vi "NavX Zero Yaw.vi"(11 "Reset NavX Yaw":bool=TRUE) -> ()   [LabVIEW 2014]
uses:
  Navx data.vi
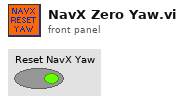
[diagram p1: front panel]
types:
  T1 = typedef "navX-MXP IMU.lvlib/navX YPRH Data.ctl" = cluster{"Yaw":dbl, "Pitch":dbl, "Roll":dbl, "Heading":dbl}
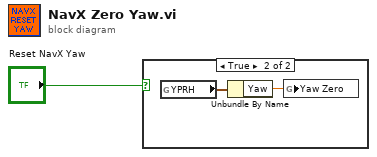
[diagram p0: block diagram]
diagram:
  n1 = case shown="True" "Reset NavX Yaw" {
    frame False {
    }
    frame True {
      n2 = global read "Navx data.vi" "YPRH"() -> (w2:T1)
      n3 = Unbundle By Name(w2) -> ("Yaw"=w3:dbl)
      n4 = global write "Navx data.vi" "Yaw Zero"(w3) -> ()
    }
  }
